vi "PPM Driver.vi"() -> ()   [LabVIEW 2021]
panel:
  out "digital waveform":digitalwaveform(waveform)={"t0"=timestamp(0 s since 1904-01-01), "dt"=1.0, "Y"={"transitions"=[], "data"=[]}}
  in  "frequency (Hz)":dbl=50.0
  in  "lines":tag="Dev1/port0/line0"
  in  "Stop Button":bool
  out "Waveform Graph":waveform(dbl)(graph)
  in  "duty cycle (%)":dbl=12.5 min=2.5 max=25.0 format="%0.2f"
  out "error out":errorcluster
  in  "Active":bool
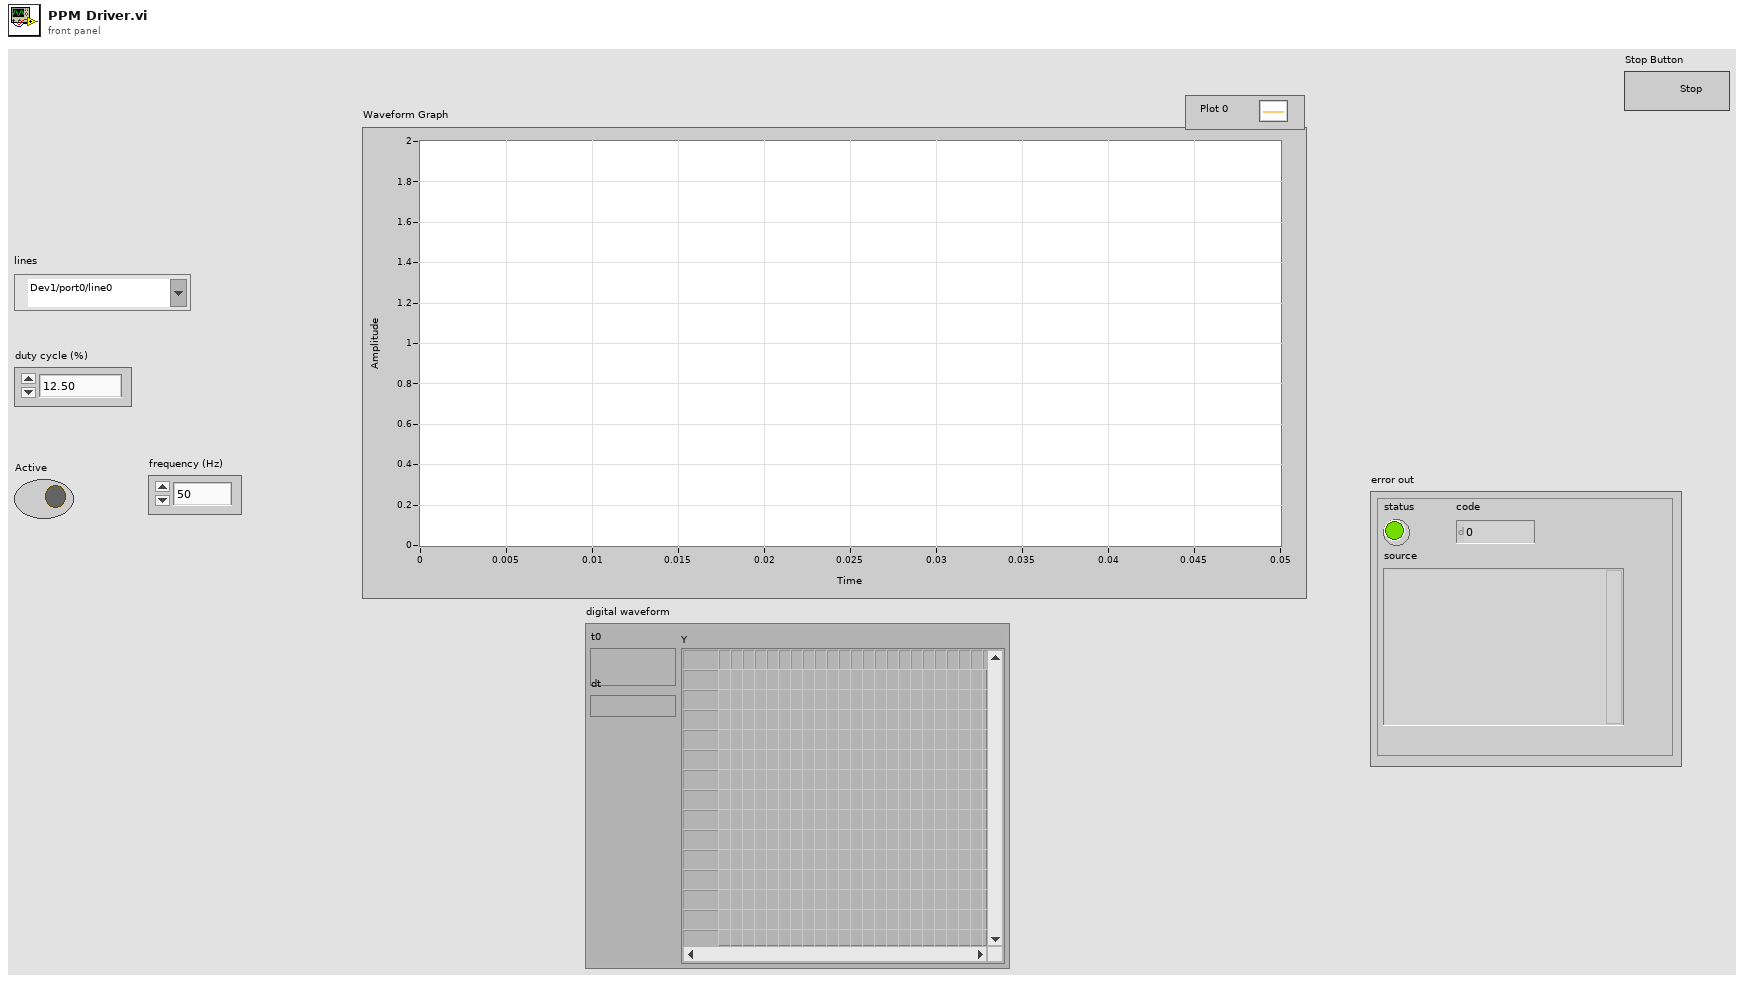
[diagram p1: front panel]
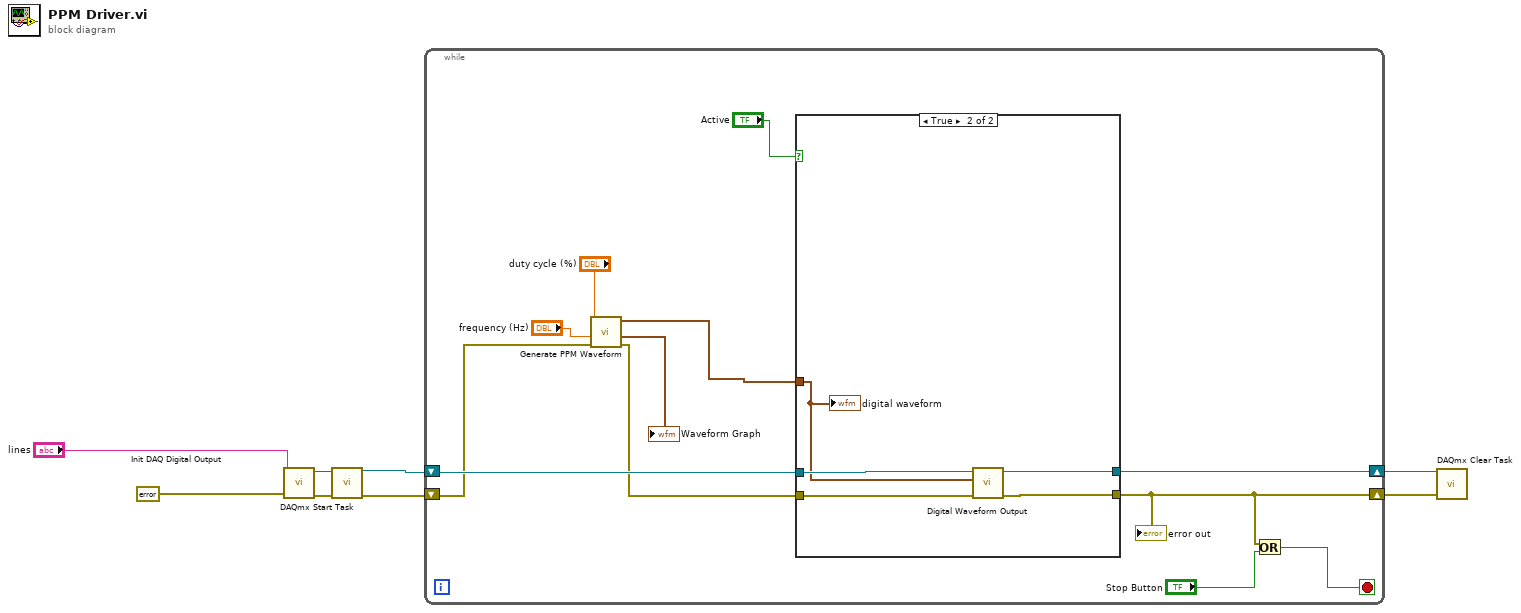
[diagram p0: block diagram]
diagram:
  n1 = call "Init DAQ Digital Output.vi"("error in"=errorcluster {"status"=FALSE, "code"=0, "source"=""}, "lines"="lines") -> ("error out"=w6:errorcluster, "Refnum out"=w7:refnum<k21>)  [unwired: 8 in]
  n2 = call <vilib>:"DAQmx Start Task.vi"("task/channels in"=w7, "error in"=w6) -> ("task out"=w5:refnum<k21>, "error out"=w4:errorcluster)  [unwired: 12 in]
  n3 = while {
    shift-right: [w10] -> w2
    shift-left: w4 -> [w15]
    shift-right: [w18] -> w3
    shift-left: w5 -> [w19]
    stop <- w11 stop-if-true
    n4 = call "Generate PPM Waveform.vi"("error in (no error)"=w15, "frequency (Hz)"="frequency (Hz)", "duty cycle (%)"="duty cycle (%)") -> ("error out"=w14:errorcluster, "Waveform Graph"=→"Waveform Graph":waveform(dbl), "digital waveform"=w17:digitalwaveform)  [unwired: 4 in, 2 out]
    n5 = case shown="True" "Active" {
      tunnel: w19 -> [w22 w27]
      tunnel: w14 -> [w21 w26]
      tunnel: [w21 w25] -> w10
      tunnel: [w22 w24] -> w18
      tunnel: w17 -> [_ w23]
      frame False {
      }
      frame True {
        n6 = call "Digital Waveform Output.vi"("error in"=w26, "Waveform"=w23, "task/channels in"=w27) -> ("error out"=w25:errorcluster, "task out"=w24:refnum<k21>)  [unwired: 7 in]
        "digital waveform" <- w23
      }
    }
    "error out" <- w10
    n7 = Or(x=w10, y="Stop Button") -> (x .or. y?=w11:bool)
  }
  n8 = call <vilib>:"DAQmx Clear Task.vi"("task in"=w3, "error in"=w2) -> ()  [unwired: 13 in, 1 out]
